vi "usermname_check.vi"(1 "first row":string[][](array[string]), 2 "String":string) -> (0 "Boolean":bool)   [LabVIEW 2014]
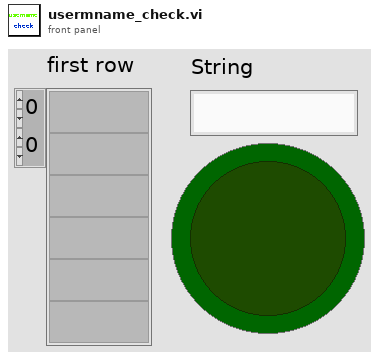
[diagram p1: front panel]
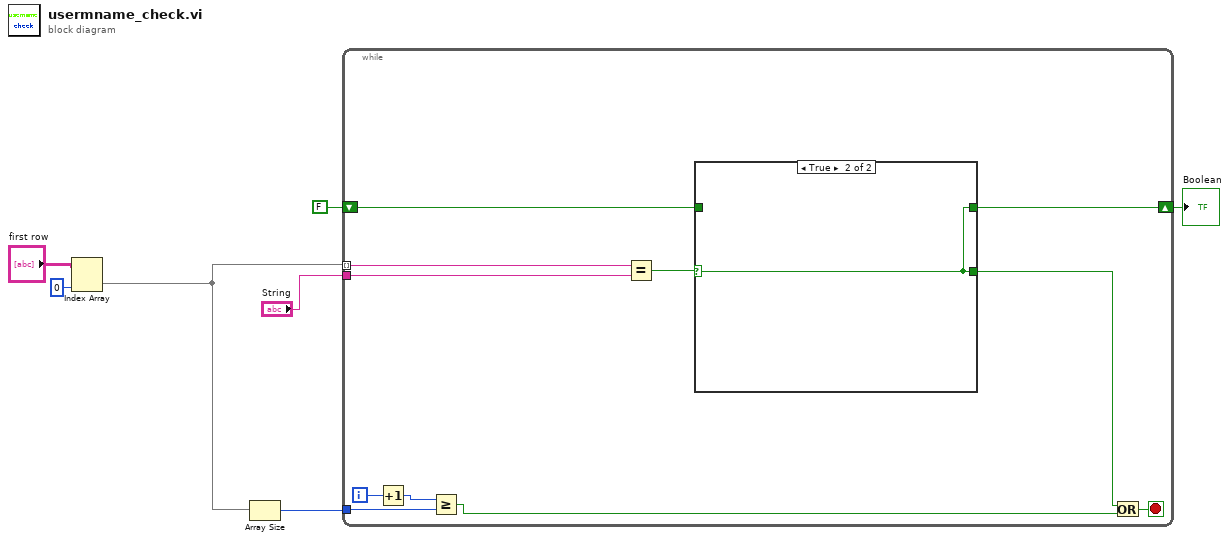
[diagram p0: block diagram]
diagram:
  n1 = Index Array(array="first row", index (col)=0 ("disabled index (col)")) -> (element=w1:string[])  [unwired: 1 in]
  n2 = Array Size(array=w1) -> (size(s)=w7:i32)
  n3 = while {
    tunnel: w7 -> [w16]
    tunnel: w1 -> [w13] mode=indexing
    tunnel: "String" -> [w12]
    shift-right: [w10] -> w4
    shift-left: FALSE -> [w9]
    i -> [w18]
    stop <- w15 stop-if-true
    n4 = Increment(x=w18) -> (x+1=w17:i32)
    n5 = Greater Or Equal?(x=w17, y=w16) -> (x >= y?=w14:bool)
    n6 = Equal?(x=w13, y=w12) -> (x = y?=w11:bool)
    n7 = case shown="True" w11 {
      selector: w11 -> [w19 w21]
      tunnel: [w20 w21] -> w10
      tunnel: w9 -> [w20 _]
      tunnel: [w19 w21] -> w8
      frame False {
      }
      frame True {
      }
    }
    n8 = Or(x=w8, y=w14) -> (x .or. y?=w15:bool)
  }
  "Boolean" <- w4
